vi "Reserve Trig0 Line.vi"(8 "error in (no error)":errorcluster) -> (0 "error out":errorcluster, 3 "Backplane refs":refnum<visa-resource-name>[](array[refnum]))   [LabVIEW 2011, in "PXIe-433x Custom Device.lvlib"]
uses:
  PXIe-433x Custom Device.lvlib
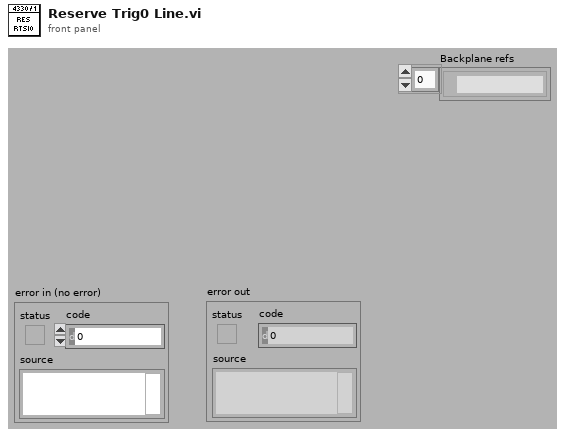
[diagram p1: front panel]
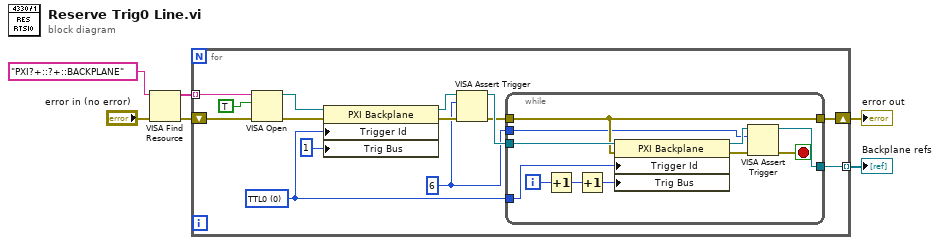
[diagram p0: block diagram]
diagram:
  n1 = VISA Find Resource(8:"error in (no error)", 11:"PXI?+::?+::BACKPLANE" ("expression (\"?*\")")) -> (0:w5:errorcluster, 3:w6:string[])  [unwired: 1 in, 1 out]
  n2 = for {
    tunnel: [w9] -> w1 mode=indexing
    shift-right: [w10] -> w2
    shift-left: w5 -> [w20]
    tunnel: w6 -> [w19] mode=indexing
    w7 = u16 6 ("protocol (default:  0)")
    w8 = i16 0 items=["Software"=-1, "TTL0"=0, "TTL1"=1, "TTL2"=2, "TTL3"=3, "TTL4"=4, "TTL5"=5, "TTL6"=6, "TTL7"=7, "ECL0"=8, "ECL1"=9] ("General Settings:Trigger Identifier")
    n3 = VISA Open(duplicate session (F)=TRUE, error in (no error)=w20, VISA resource name=w19) -> (VISA resource name=w16:refnum<visa-resource-name>, error out=w17:errorcluster)  [unwired: 2 in]
    n4 = property class="PXI Backplane"(reference=w16, error in=w17, "Trigger Id"=w8, "Trig Bus"=i16 1 ("PXI/PCI Settings:Trigger Bus Number")) -> (reference out=w13:refnum<visa-resource-name>, error out=w14:errorcluster)
    n5 = VISA Assert Trigger(8:w14, 10:w7, 11:w13) -> (0:w11:errorcluster, 3:w12:refnum<visa-resource-name>)
    n6 = while {
      tunnel: [w28] -> w10
      tunnel: w12 -> [w31]
      tunnel: w11 -> [w28]
      tunnel: [w24] -> w9
      tunnel: w8 -> [w23]
      tunnel: w7 -> [w22]
      i -> [w30]
      stop <- w25 stop-if-true
      n7 = Increment(x=w30) -> (x+1=w21:i32)
      n8 = Increment(x=w21) -> (x+1=w29:i32)
      n9 = property class="PXI Backplane"(reference=w31, error in=w28, "Trigger Id"=w23, "Trig Bus"=w29) -> (reference out=w26:refnum<visa-resource-name>, error out=w27:errorcluster)
      n10 = VISA Assert Trigger(8:w27, 10:w22, 11:w26) -> (0:w25:errorcluster, 3:w24:refnum<visa-resource-name>)
    }
  }
  "error out" <- w2
  "Backplane refs" <- w1
